vi "reconnect.vi"(8 "error in (no error)":errorcluster, 11 "TCPCommunicator in":refnum<class "TCPCommunicator.lvclass">) -> (0 "error out":errorcluster, 3 "TCPCommunicator out":refnum<class "TCPCommunicator.lvclass">)   [LabVIEW 2016, in "TCPCommunicator.lvclass"]
uses:
  TCPCommunicator.lvclass
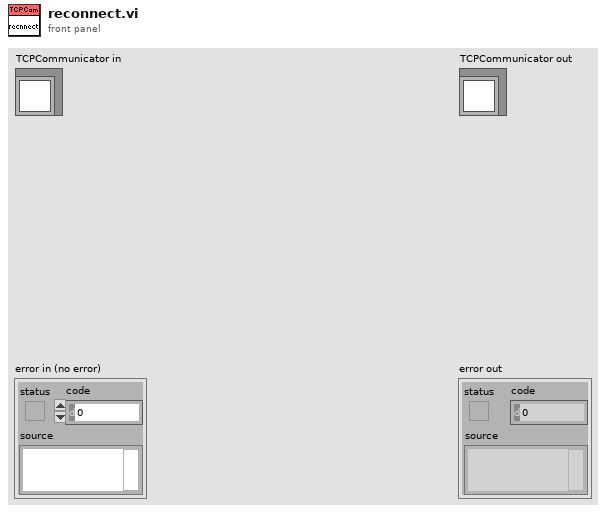
[diagram p1: front panel]
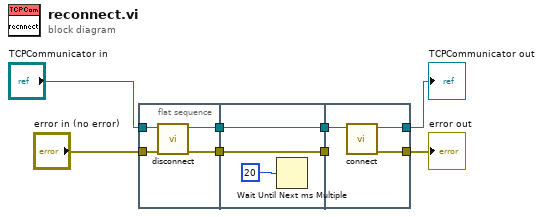
[diagram p0: block diagram]
diagram:
  n1 = flat-sequence {
    tunnel: [w11] -> w8
    tunnel: "error in (no error)" -> [w12]
    tunnel: "TCPCommunicator in" -> [w10]
    tunnel: [w9] -> w7
    tunnel: w8 -> [w13]
    tunnel: [w14] -> w6
    tunnel: w7 -> [w14]
    tunnel: [w13] -> w5
    tunnel: [w18] -> w1
    tunnel: w6 -> [w17]
    tunnel: w5 -> [_]
    tunnel: [w16] -> w2
    frame #0 {
      n2 = call-dynamic "disconnect.vi"("error in (no error)"=w12, "TCPCommunicator in"=w10) -> ("error out"=w11:errorcluster, "TCPCommunicator out"=w9:refnum<class "TCPCommunicator.lvclass">)  [unwired: 8 in]
    }
    frame #1 {
      n3 = Wait Until Next ms Multiple(millisecond multiple=20) -> ()  [unwired: 1 out]
    }
    frame #2 {
      n4 = call-dynamic "connect.vi"("TCPCommunicator in"=w17) -> ("error out"=w18:errorcluster, "TCPCommunicator out"=w16:refnum<class "TCPCommunicator.lvclass">)  [unwired: 9 in]
    }
  }
  "error out" <- w1
  "TCPCommunicator out" <- w2
